vi "Actor Core.vi"(8 "error in":errorcluster, 11 "Mediator in":refnum<class "Mediator.lvclass">) -> (0 "error out":errorcluster, 3 "Actor out":refnum<class "Actor.lvclass">)   [LabVIEW 2015, in "Mediator.lvlib" / "Mediator.lvclass"]
doc: "(<B>Filename</B>: Actor Framework.lvlib:Actor.lvclass:Actor Core.vi)\n\nReceives messages to the actor, reacts to them, and initiates any error handling that may shut the actor down.\n\nDescendant classes may override this VI to append parallel tasks for the actor to complete while it handles messages. Overrides use the Call Parent Method node."
uses:
  Mediator.lvclass
  <vilib>/ActorFramework/Actor/Actor.lvclass
  Mediator.lvclass/Mediator.ctl
  IMediator/IMediator/IMediator.lvclass
panel:
  in  "TopicTree":string[](tree)
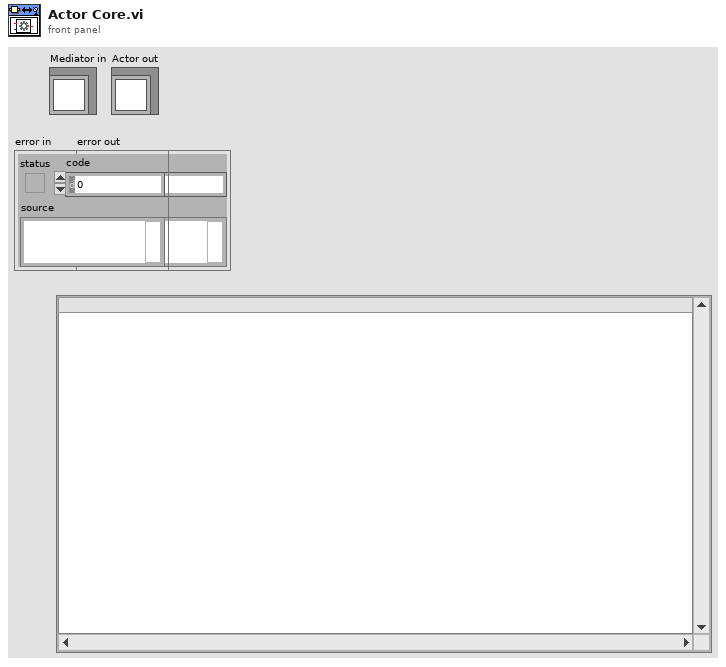
[diagram p1: front panel]
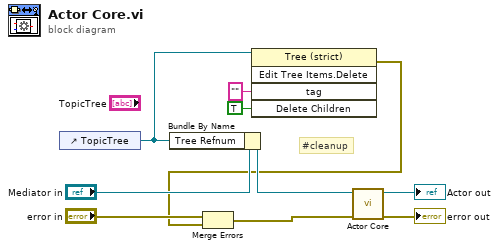
[diagram p0: block diagram]
diagram:
  # "#cleanup"
  n1 = control-ref of="TopicTree"() -> (w5:refnum<vi>)
  n2 = Bundle By Name(cluster="Mediator in", "Tree Refnum"=w5) -> (w6:refnum<class "Mediator.lvclass">)
  n3 = invoke class="Tree (strict)" method="Edit Tree Items.Delete"(reference=w5, "tag"="" ("Tag"), "Delete Children"=TRUE ("Delete Children?")) -> (error out=w1:errorcluster)  [unwired: 2 in, 4 out]
  n4 = Merge Errors("error in", w1) -> (w2:errorcluster)
  n5 = call-parent "Actor Core.vi"("error in"=w2, "Actor in"=w6) -> ("error out"=→"error out":errorcluster, "Actor out"=→"Actor out":refnum<class "Actor.lvclass">)  [unwired: 8 in]
